vi "Shutdown.vi"(8 "error in (no error)":errorcluster, 11 "UDP Transceiver in":refnum<class "UDP Transceiver.lvclass">=refnum) -> (0 "error out":errorcluster, 3 "UDP Transceiver out":refnum<class "UDP Transceiver.lvclass">)   [LabVIEW 2020, in "UDP.lvlib" / "UDP Transceiver.lvclass"]
uses:
  UDP Transceiver.lvclass
  Transfer Parameters.ctl
  Transfer Group Parameters.ctl
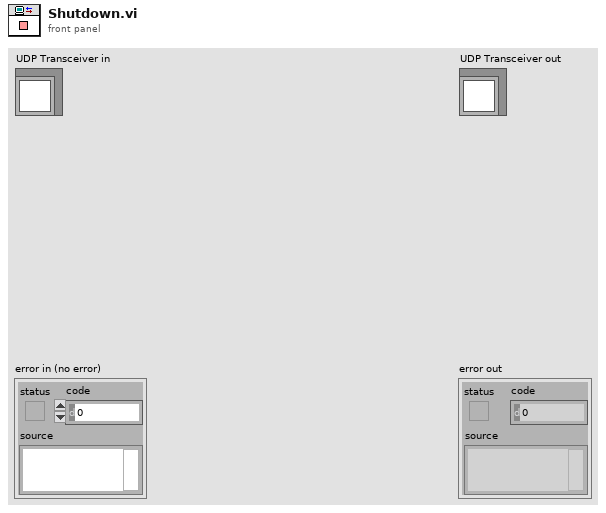
[diagram p1: front panel]
types:
  T1 = typedef "UDP.lvlib/UDP Transceiver.lvclass/Transfer Group Parameters.ctl" = cluster{"transfers":T2[], "max size":i32, "timeout":i32}
  T2 = typedef "UDP.lvlib/UDP Transceiver.lvclass/Transfer Parameters.ctl" = cluster{"group offset":u64, "size":u64, "address":u32, "port":u16}
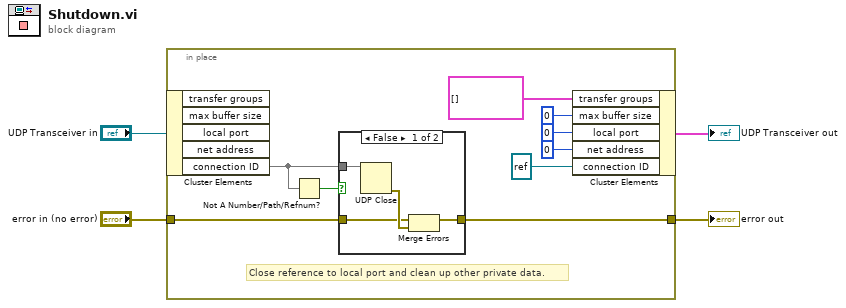
[diagram p0: block diagram]
diagram:
  n1 = in-place {
    in-place-border: "error in (no error)" -> [w13]
    in-place-border: [w12] -> w3
    # "Close reference to local port and clean up other private data."
    n2 = in-place-cluster #1("UDP Transceiver in") -> ("connection ID"=w11)  [unwired: 4 out]
    n3 = Not A Number/Path/Refnum?(number/path/refnum=w11) -> (NaN/Path/Refnum?=w10:bool)
    n4 = case shown="False" w10 {
      tunnel: w13 -> [w16 w18]
      tunnel: [w15 w18] -> w12
      tunnel: w11 -> [w14 _]
      frame False {
        n5 = UDP Close(connection ID=w14) -> (error out=w17:errorcluster)  [unwired: 1 in, 1 out]
        n6 = Merge Errors(w16, w17) -> (w15:errorcluster)
      }
      frame True {
      }
    }
    n7 = in-place-cluster #1("transfer groups"=T1[] [] ("Transfer Group parameters"), "max buffer size"=u64 0, "local port"=u16 0, "net address"=u32 0, "connection ID"=refnum<k16> refnum ("connection ID out")) -> (→"UDP Transceiver out":cluster{})
  }
  "error out" <- w3
